vi "Abort VI.vi"() -> ()   [LabVIEW 2019]
panel:
  in  "VI name":string="Batch Load Data.vi"
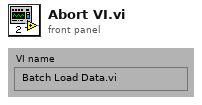
[diagram p1: front panel]
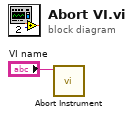
[diagram p0: block diagram]
diagram:
  n1 = call <vilib>:"Abort Instrument.vi"("VI name"="VI name") -> ()  [unwired: 10 in, 1 out]
